vi "Write SerialNumber.vi"(8 "error in (no error)":errorcluster, 10 "SerialNumber":string, 11 "UnitTestEngine in":refnum<class "UnitTestEngine.lvclass">) -> (0 "error out":errorcluster, 3 "UnitTestEngine out":refnum<class "UnitTestEngine.lvclass">)   [LabVIEW 2019, in "UnitTestEngine.lvlib" / "UnitTestEngine.lvclass"]
uses:
  UnitTestEngine.lvclass
  UnitTestEngine.lvclass/UnitTestEngine.ctl
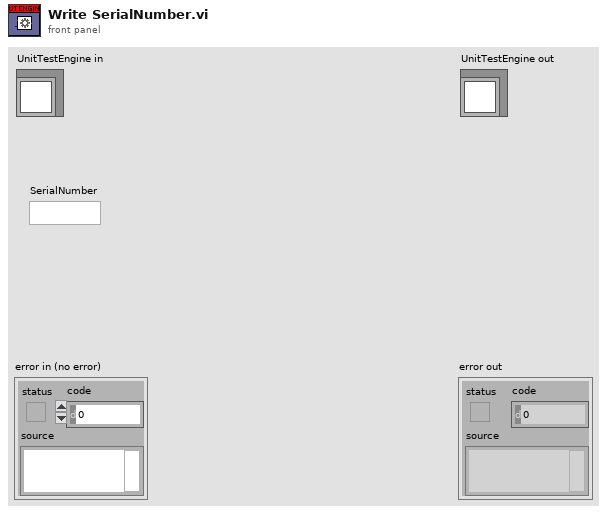
[diagram p1: front panel]
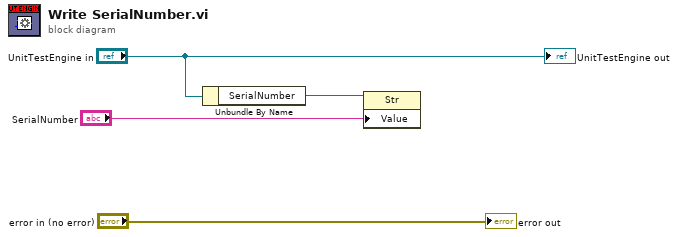
[diagram p0: block diagram]
diagram:
  n1 = Unbundle By Name("UnitTestEngine in") -> ("SerialNumber"=w2:refnum<vi>)
  n2 = property class="Str"(reference=w2, "Value"="SerialNumber") -> ()  [unwired: 1 in, 2 out]
  "error out" <- "error in (no error)"
  "UnitTestEngine out" <- "UnitTestEngine in"
